vi "ConvertPathsToStrings.vi"(6 "Show full paths":bool, 10 "header files in":path[](array[path])) -> (3 "header files str":string[](array[string]))   [LabVIEW 2016]
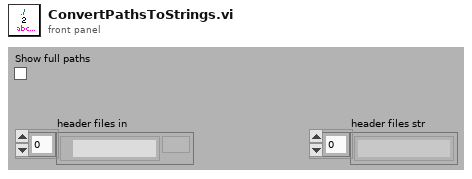
[diagram p1: front panel]
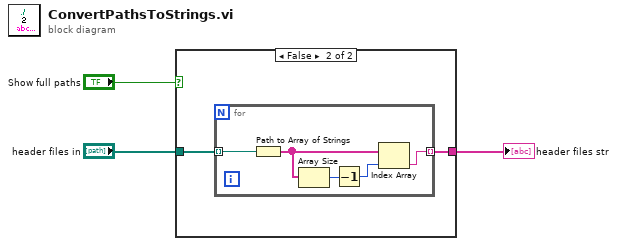
[diagram p0: block diagram]
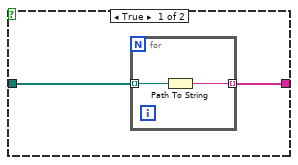
[diagram p2: hidden frame]
diagram:
  n1 = case shown="False" "Show full paths" {
    tunnel: "header files in" -> [w5 w9]
    tunnel: [w4 w8] -> w2
    frame True {
      n2 = for {
        tunnel: w5 -> [w7] mode=indexing
        tunnel: [w6] -> w4 mode=indexing
        n3 = Path To String(path=w7) -> (string=w6:string)
      }
    }
    frame False {
      n4 = for {
        tunnel: w9 -> [w14] mode=indexing
        tunnel: [w13] -> w8 mode=indexing
        n5 = Path to Array of Strings(0:w14) -> (2:w11:string[])  [unwired: 1 out]
        n6 = Array Size(array=w11) -> (size(s)=w12:i32)
        n7 = Decrement(x=w12) -> (x-1=w10:i32)
        n8 = Index Array(array=w11, index=w10) -> (element=w13:string)
      }
    }
  }
  "header files str" <- w2
